vi "LVClass_Pupil Save Data.vi"(0 "Pupil in":refnum<class "Pupil.lvclass">, 11 "error in (no error)":errorcluster) -> (4 "Pupil out":refnum<class "Pupil.lvclass">, 15 "error out":errorcluster)   [LabVIEW 2020, in "Pupil.lvclass"]
uses:
  Pupil.lvclass
  Pupil.lvclass/Pupil.ctl
panel:
  in  "Path (dialog if empty)":path
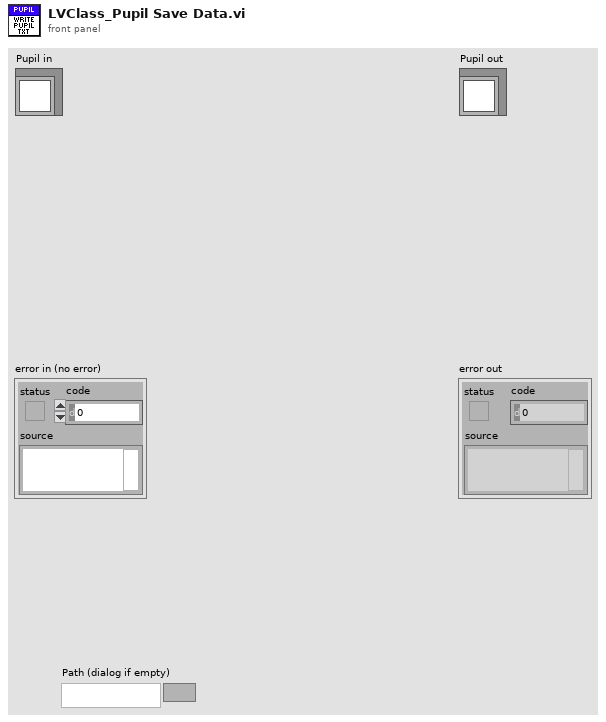
[diagram p1: front panel]
types:
  T1 = typedef "ClassID.ctl" = i64
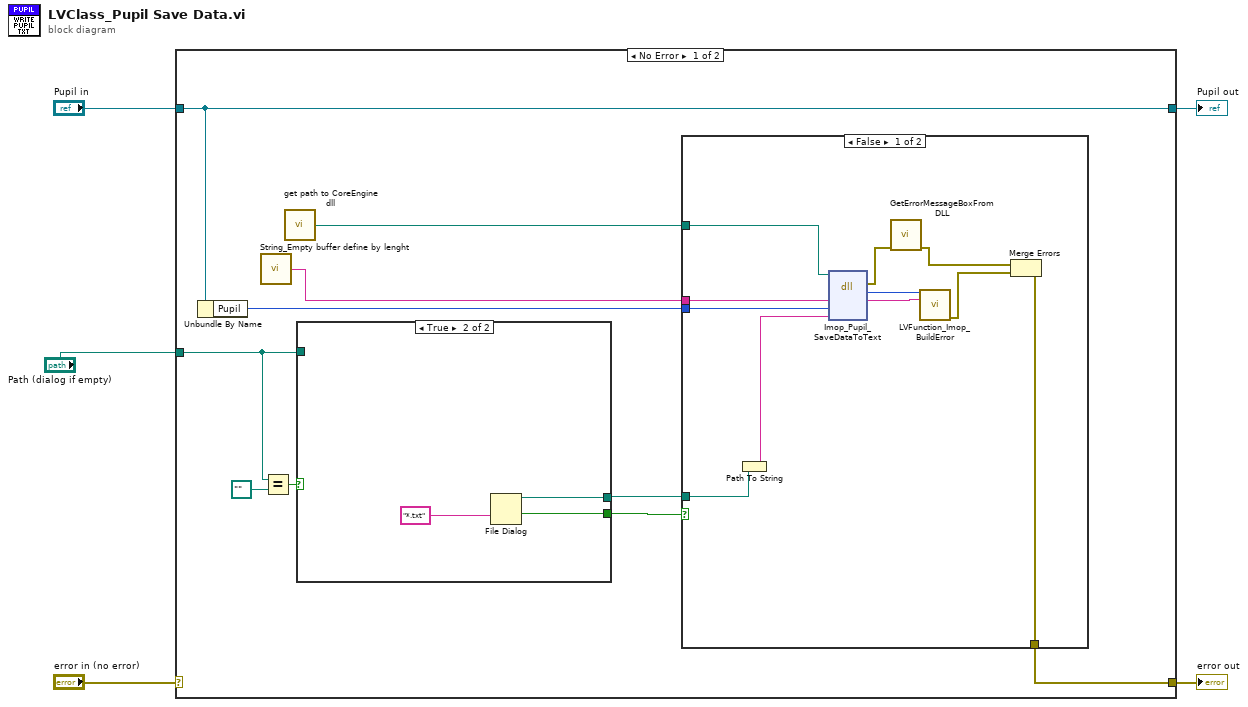
[diagram p0: block diagram]
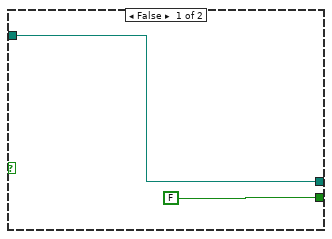
[diagram p3: hidden frame]
diagram:
  n1 = case shown="No Error" "error in (no error)" {
    selector: "error in (no error)" -> [_ w33]
    tunnel: [w11 w33] -> w4
    tunnel: [w12 w32] -> w2
    tunnel: "Pupil in" -> [w12 w32]
    tunnel: "Path (dialog if empty)" -> [w6 _]
    frame No Error {
      n2 = Unbundle By Name(w12) -> ("Pupil"=w13:T1)
      n3 = call "String_Empty buffer define by lenght.vi"() -> ("Empty buffer"=w15:string)  [unwired: 1 in]
      n4 = Equal?(x=w6, y=path "") -> (x = y?=w10:bool)
      n5 = call "get path to CoreEngine dll.vi"() -> ("path to wavekit library"=w14:path)  [unwired: 14 in, 1 out]
      n6 = case shown="True" w10 {
        tunnel: [w27 w31] -> w8
        tunnel: w6 -> [w27 _]
        tunnel: [FALSE ("cancelled") w30] -> w7
        frame False {
        }
        frame True {
          n7 = File Dialog(6:"*.txt" ("pattern")) -> (1:w30:bool, 3:w31:path)  [unwired: 6 in, 2 out]
        }
      }
      n8 = case shown="False" w7 {
        tunnel: w15 -> [w26 _]
        tunnel: w14 -> [w23 _]
        tunnel: w13 -> [w21 _]
        tunnel: [w18 _] -> w11
        tunnel: w8 -> [w17 _]
        frame False {
          n9 = Path To String(path=w17) -> (string=w16:string)
          n10 = dll-call lib="D:/2_trunk/Soft_haso/ImOpCoreEngine4_LV2011/DLLs/ImopEngine4_vc100.dll" fn="Imop_Pupil_SaveDataToText"(path in=w23, "message"=w26, "objet"=w21, "Data"=w16) -> (error out=w22:errorcluster, "return type"=w24:i32, "message"=w25:string)  [unwired: 4 in, 1 out]
          n11 = call "GetErrorMessageBoxFromDLL.vi"("error IN"=w22) -> ("error OUT"=w20:errorcluster)  [unwired: 10 in]
          n12 = call "LVFunction_Imop_BuildError.vi"("code"=w24, "String to Prepend to source (\"\")"=w25) -> ("error out"=w19:errorcluster)  [unwired: 13 in]
          n13 = Merge Errors(w20, w19) -> (w18:errorcluster)
        }
        frame True {
        }
      }
    }
    frame Error {
    }
  }
  "error out" <- w4
  "Pupil out" <- w2
